vi "Clear Modify Object Before.vi"(8 "error in (no error)":errorcluster, 11 "Canvas in":refnum<class "Canvas.lvclass">) -> (0 "error out":errorcluster, 2 "ID":i32, 3 "Canvas out":refnum<class "Canvas.lvclass">)   [LabVIEW 2015, in "Canvas.lvclass"]
uses:
  Canvas.lvclass
  Canvas.lvclass/Canvas.ctl
  Graphic/Graphic.lvclass/Graphic.ctl
  Graphic/Graphic.lvclass
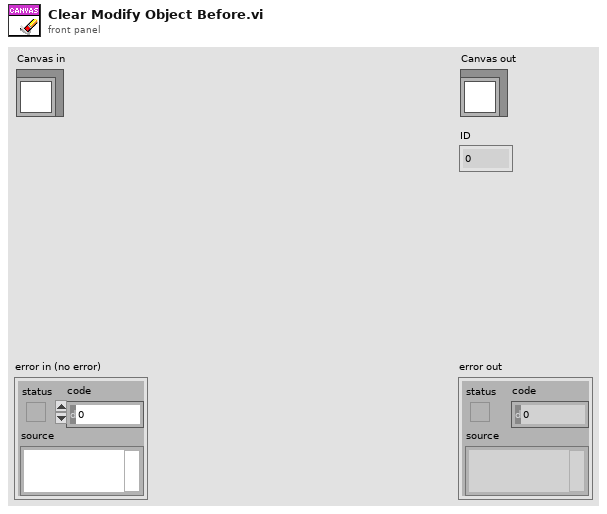
[diagram p1: front panel]
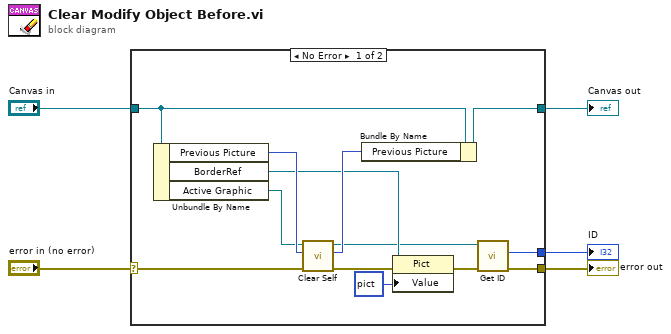
[diagram p0: block diagram]
diagram:
  n1 = case shown="No Error" "error in (no error)" {
    selector: "error in (no error)" -> [w14 w20]
    tunnel: [w8 w20] -> w4
    tunnel: [w16 w19] -> w2
    tunnel: "Canvas in" -> [w18 w19]
    tunnel: [w6 _] -> w1
    frame No Error {
      n2 = Unbundle By Name(w18) -> ("Previous Picture"=w17:picture, "BorderRef"=w13:refnum<vi>, "Active Graphic"=w10:refnum<class "Graphic.lvclass">)
      n3 = call-dynamic "Clear Self.vi"("error in (no error)"=w14, "Picture in"=w17, "Graphic in"=w10) -> ("error out"=w11:errorcluster, "Picture out"=w15:picture, "Graphic out"=w7:refnum<class "Graphic.lvclass">)  [unwired: 6 in]
      n4 = Bundle By Name(cluster=w18, "Previous Picture"=w15) -> (w16:refnum<class "Canvas.lvclass">)
      n5 = property class="Pict"(reference=w13, error in=w11, "Value"=picture data[5B]) -> (error out=w9:errorcluster)  [unwired: 1 out]
      n6 = call "Get ID.vi"("error in (no error)"=w9, "Graphic in"=w7) -> ("error out"=w8:errorcluster, "ID"=w6:i32)  [unwired: 7 in, 1 out]
    }
    frame Error {
    }
  }
  "error out" <- w4
  "Canvas out" <- w2
  "ID" <- w1
